vi "Find_calibration_file.vi"(1 "Inst type":T1=enum."Pressure Transducer", 2 "Channel ID":string, 3 "Use Latest Calib":bool, 4 "filename":path) -> (0 "filename out":path)   [LabVIEW 2017]
uses:
  Controls/Inst_type.ctl
  Controls/App_Global.ctl
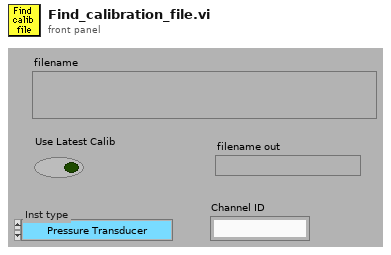
[diagram p1: front panel]
types:
  T1 = typedef "Inst_type.ctl" = enum16{"Propeller anemometer", "Raw voltage", "Pressure Transducer", "Pitot-static tube", "Preston tube", "Hot wire", "Cross wire 1", "Cross wire 2", "Generic Linear", "Generic Polynomial", "Generic BackPoly", "Fast FID", "Thermocouple", "Cold wire", "Pulsed Wire", "LDA Vel", "LDA Tran time", "LDA Arr time", "Microphone"}
  T2 = typedef "App_Global.ctl" = enum16{"Read Global", "Write to Global", "Initialise Array"}
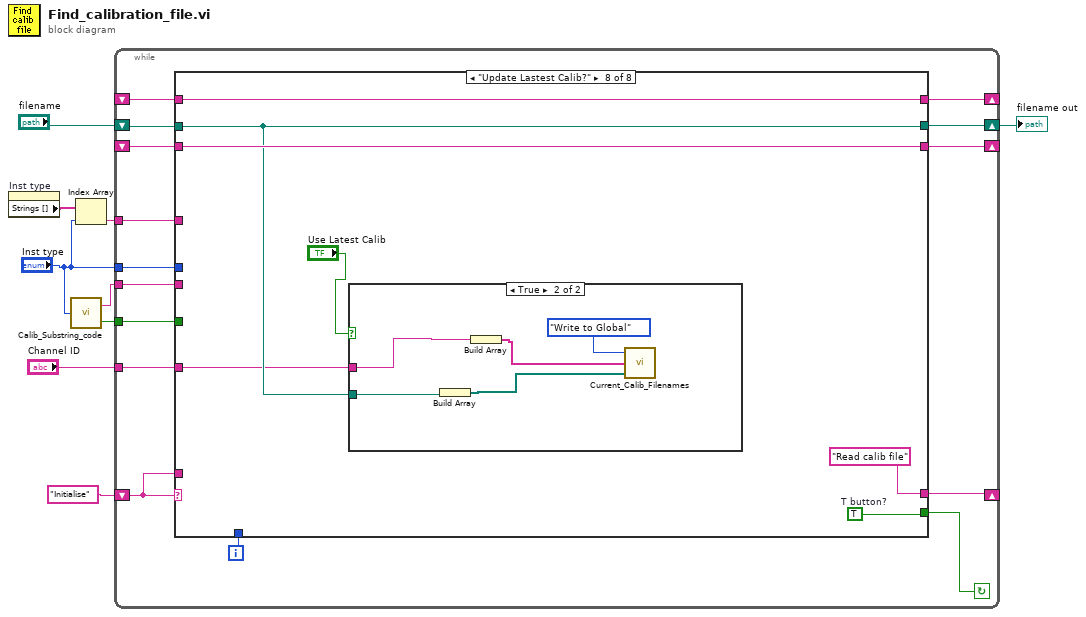
[diagram p0: block diagram]
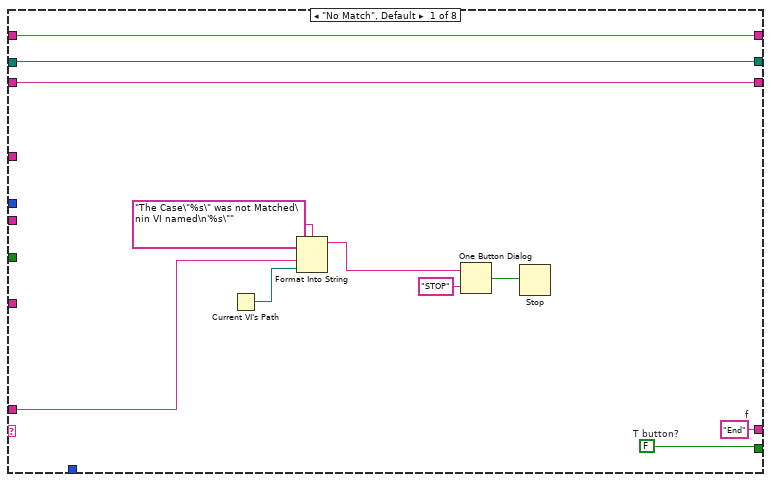
[diagram p2: hidden frame]
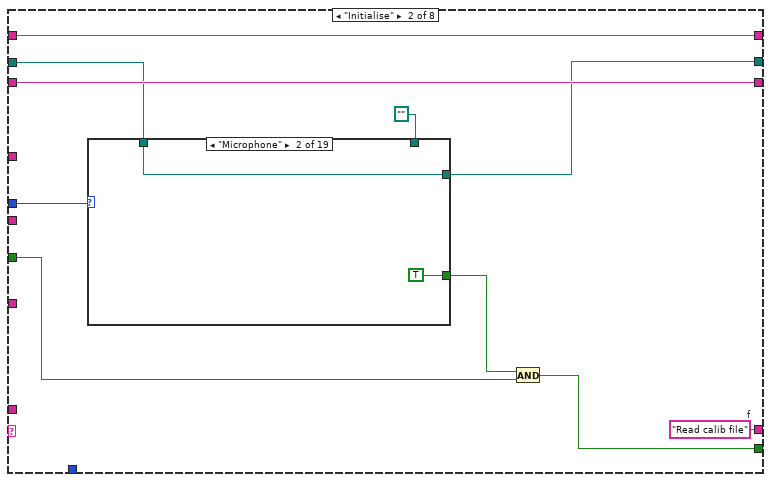
[diagram p3: hidden frame]
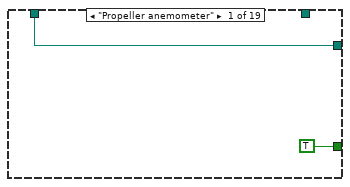
[diagram p4: hidden frame]
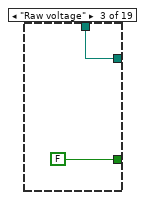
[diagram p5: hidden frame]
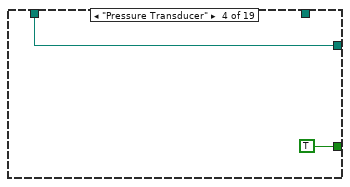
[diagram p6: hidden frame]
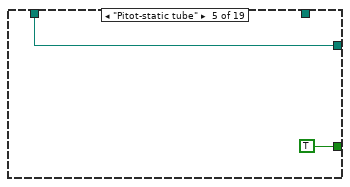
[diagram p7: hidden frame]
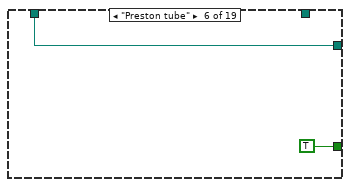
[diagram p8: hidden frame]
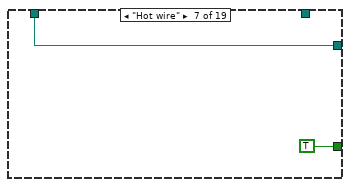
[diagram p9: hidden frame]
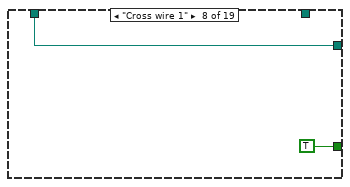
[diagram p10: hidden frame]
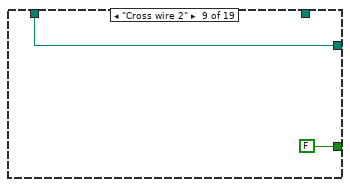
[diagram p11: hidden frame]
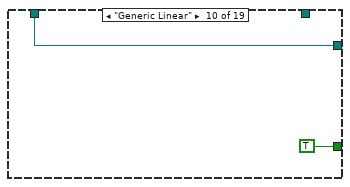
[diagram p12: hidden frame]
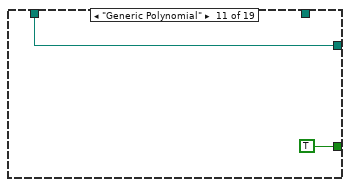
[diagram p13: hidden frame]
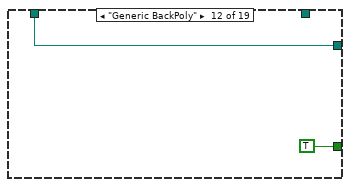
[diagram p14: hidden frame]
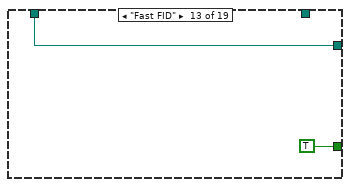
[diagram p15: hidden frame]
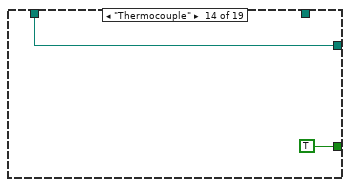
[diagram p16: hidden frame]
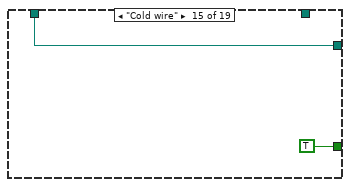
[diagram p17: hidden frame]
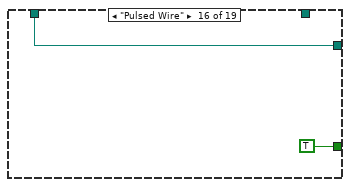
[diagram p18: hidden frame]
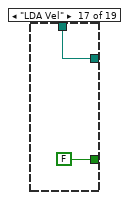
[diagram p19: hidden frame]
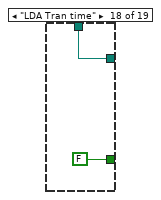
[diagram p20: hidden frame]
diagram:
  n1 = property on="Inst type" class="Enum (strict)"() -> ("Strings []"=w6:string[])  [unwired: 2 in, 2 out]
  n2 = call "Calib_Substring_code.vi"("Inst type"="Inst type") -> ("Substring Type"=w3:string, "Read file"=w2:bool)
  n3 = Index Array(array=w6, index="Inst type") -> (element=w5:string)
  n4 = while {
    shift-left: "filename" -> [w24]
    shift-right: [w23] -> w8
    shift-left: "Initialise" -> [w17]
    shift-right: [w22] -> _
    shift-right: [w19] -> _
    shift-left: _ -> [w18]
    tunnel: "Inst type" -> [w16]
    tunnel: w5 -> [w15]
    shift-right: [w13] -> _
    shift-left: _ -> [w14]
    tunnel: w3 -> [w12]
    tunnel: w2 -> [w11]
    tunnel: "Channel ID" -> [w10]
    i -> [w20]
    stop <- w21 continue-if-true
    n5 = case shown="\"Update Lastest Calib?\"" w17 {
      tunnel: w24 -> [w34 w40 w91 w97 w107 w129 w162 w191]
      tunnel: [w34 w41 w91 w94 w107 w129 w162 w191] -> w23
      tunnel: [w33 w42 w87 "Update Lastest Calib?" w112 w141 "Find a Calibration file" "Read calib file" ("f")] -> w22
      tunnel: [w32 w36 TRUE w103 w115 w142 w177 w189] -> w21
      tunnel: w20 -> [_ _ _ _ _ _ _ _]
      tunnel: [w35 w45 w86 w105 w110 w139 w164 w193] -> w19
      tunnel: w18 -> [w35 w45 _ w105 w110 w139 w164 w193]
      tunnel: w17 -> [w26 _ _ _ _ _ _ _]
      tunnel: w16 -> [_ w43 _ _ _ w140 _ _]
      tunnel: w15 -> [_ _ _ w101 w113 _ _ _]
      tunnel: w14 -> [w25 w44 w84 w102 _ w138 w165 w192]
      tunnel: [w25 w44 w84 w102 w111 w138 w165 w192] -> w13
      tunnel: w12 -> [_ _ _ _ w109 _ _ _]
      tunnel: w11 -> [_ w37 _ _ _ _ _ _]
      tunnel: w10 -> [_ _ _ w99 _ _ _ w188]
      frame "No Match", Default {
        w32 = FALSE  # T button?
        w33 = "End"  # f
        n6 = Current VI's Path() -> (path=w27:path)
        n7 = Format Into String(format string="The Case\"%s\" was not Matched\nin VI named\n'%s\"" ("Format String"), w26, w27) -> (resulting string=w30:string)  [unwired: 2 in, 1 out]
        n8 = One Button Dialog(message=w30, button name ("OK")="STOP") -> (true=w28:bool)
        n9 = Stop(stop? (T)=w28) -> ()
      }
      frame "Initialise" {
        w42 = "Read calib file"  # f
        n10 = case shown="\"Microphone\"" w43 {
          tunnel: [TRUE TRUE FALSE TRUE TRUE TRUE TRUE TRUE FALSE TRUE TRUE TRUE TRUE TRUE TRUE TRUE FALSE FALSE FALSE] -> w38
          tunnel: [w46 w48 w50 w52 w54 w56 w58 w60 w62 w64 w66 w68 w70 w72 w74 w76 w78 w80 w82] -> w41
          tunnel: w40 -> [w46 w48 _ w52 w54 w56 w58 w60 w62 w64 w66 w68 w70 w72 w74 w76 _ _ _]
          tunnel: path "" -> [_ _ w50 _ _ _ _ _ _ _ _ _ _ _ _ _ w78 w80 w82]
          frame "Propeller anemometer" {
          }
          frame "Microphone" {
          }
          frame "Raw voltage" {
          }
          frame "Pressure Transducer" {
          }
          frame "Pitot-static tube" {
          }
          frame "Preston tube" {
          }
          frame "Hot wire" {
          }
          frame "Cross wire 1" {
          }
          frame "Cross wire 2" {
          }
          frame "Generic Linear" {
          }
          frame "Generic Polynomial" {
          }
          frame "Generic BackPoly" {
          }
          frame "Fast FID" {
          }
          frame "Thermocouple" {
          }
          frame "Cold wire" {
          }
          frame "Pulsed Wire" {
          }
          frame "LDA Vel" {
          }
          frame "LDA Tran time" {
          }
          frame "LDA Arr time" {
          }
        }
        n11 = And(x=w38, y=w37) -> (x .and. y?=w36:bool)
      }
      frame "Read calib file" {
        w85 = "Check for calib substring"  # f
        n12 = call "Read_File_Simple.vi"("Filename"=w91) -> ("Error?"=w89:bool, "string"=w86:string)  [unwired: 2 in, 6 out]
        n13 = Select(t="Find a Calibration file", s=w89, f=w85) -> (s? t:f=w87:string)
      }
      frame "Find a Calibration file" {
        n14 = Format Into String(format string=" calibration file for channel %s not found.  Please search for it.", initial string=w101, w99) -> (resulting string=w93:string)  [unwired: 1 in, 1 out]
        n15 = call "Current_Filepath.vi"("Short_Name"="Cal" ("Data Type"), "Filename in"=w97, "Data Type"="Calibrations") -> ("Directory"=w96:path)  [unwired: 1 in, 1 out]
        n16 = call "File Dialog"("start path"=w96, "prompt"=w93) -> ("selected path"=w94:path, "cancelled"=w95:bool)  [unwired: 10 in, 2 out]
        n17 = Not(x=w95) -> (.not. x?=w103:bool)
      }
      frame "Check for calib substring" {
        w117 = FALSE  # Show Dialog?
        n18 = Concatenate Strings(w109, "calib label") -> (w114:string)
        n19 = Format Into String(format string="Calibration File   %s", w107) -> (resulting string=w106:string)  [unwired: 2 in, 1 out]
        n20 = call "Get_string_subset.vi"("String Name"=w106, "Show Dialog?"=w117, "String to split"=w110, "File Label"=w114) -> ("Status"=w116:enum16{"Char in string", "Char not in string"}, "Output string"=w111:string)
        n21 = case shown="\"Char in string\"" w116 {
          tunnel: [TRUE w126] -> w115
          tunnel: w107 -> [_ w122]
          tunnel: w113 -> [_ w125]
          tunnel: ["Was there sufficient calibration points?" "Find a Calibration file"] -> w112
          frame "Char in string" {
          }
          frame "Char not in string" {
            w123 = "The calibration file\n\"%s\"\nis not the appropriate file for a %s"  # format string
            w127 = "Find another file"  # T button name ("OK")
            n22 = Strip Path(path=w122) -> (name=w121:string)  [unwired: 1 out]
            n23 = Format Into String(format string=w123, w121, w125) -> (resulting string=w128:string)  [unwired: 2 in, 1 out]
            n24 = Two Button Dialog(message=w128, 2:w127) -> (T button?=w126:bool)  [unwired: 1 out]
          }
        }
      }
      frame "Was there sufficient calibration points?" {
        n25 = Format Into String(format string="Calibration File   %s", w129) -> (resulting string=w130:string)  [unwired: 2 in, 1 out]
        n26 = call "2D_array_from_string.vi"("String Name"=w130, "Input string"=w138, "Array title"="Calib points label") -> ("2D data array"=w137:dbl[][])  [unwired: 1 in]
        n27 = for {
          tunnel: w137 -> [w148] mode=indexing
          tunnel: [w144] -> w133 mode=indexing
          n28 = Index Array(array=w148, index=5) -> (element=w146:dbl)
          n29 = Not A Number/Path/Refnum?(number/path/refnum=w146) -> (NaN/Path/Refnum?=w145:bool)
          n30 = Not(x=w145) -> (.not. x?=w144:bool)
        }
        n31 = Boolean To (0,1)(Boolean=w133) -> (0, 1=w136:i16[])
        n32 = Add Array Elements(numeric array=w136) -> (sum=w134:i16)
        n33 = Greater?(x=w134, y=i16 1) -> (0:w132:bool)
        n34 = case shown="True" w132 {
          tunnel: [w153 w157] -> w142
          tunnel: w129 -> [w150 _]
          tunnel: ["Find a Calibration file" "Are XW psi 1 and 2 valid"] -> w141
          tunnel: w140 -> [_ w158]
          frame False {
            w151 = "The calibration file\n\"%s\"\nhas less than two calibration points."  # format string
            w154 = "Find another file"  # T button name ("OK")
            n35 = Strip Path(path=w150) -> (name=w149:string)  [unwired: 1 out]
            n36 = Format Into String(format string=w151, w149) -> (resulting string=w155:string)  [unwired: 2 in, 1 out]
            n37 = Two Button Dialog(message=w155, 2:w154) -> (T button?=w153:bool)  [unwired: 1 out]
          }
          frame True {
            n38 = case shown="\"Propeller anemometer\", Default" w158 {
              tunnel: [FALSE TRUE] -> w157
              frame "Propeller anemometer", Default {
              }
              frame "Cross wire 1" {
              }
            }
          }
        }
      }
      frame "Are XW psi 1 and 2 valid" {
        w170 = FALSE  # Show Dialog?
        n39 = Build Array("C0", "C1", "C2") -> (w172:string[])
        n40 = Format Into String(format string="Calibration File   %s", w162) -> (resulting string=w161:string)  [unwired: 2 in, 1 out]
        n41 = call "Get_string_subset.vi"("String Name"=w161, "Show Dialog?"=w170, "String to split"=w164, "File Label"="Auxiliary constants") -> ("Output string"=w171:string)  [unwired: 1 out]
        n42 = for {
          tunnel: w172 -> [w180] mode=indexing
          tunnel: [w179] -> w169 mode=indexing
          tunnel: w171 -> [w178]
          n43 = call "Get_value_from_string.vi"("Input string"=w178, "Variable name"=w180) -> ("Value"=w179:dbl)  [unwired: 1 in, 1 out]
        }
        n44 = Not A Number/Path/Refnum?(number/path/refnum=w169) -> (NaN/Path/Refnum?=w168:bool[])
        n45 = Or Array Elements(Boolean array=w168) -> (logical OR=w167:bool)
        n46 = case shown="False" w167 {
          tunnel: [FALSE w185] -> w177
          tunnel: w162 -> [_ w183]
          frame False {
          }
          frame True {
            n47 = Strip Path(path=w183) -> (name=w182:string)  [unwired: 1 out]
            n48 = Format Into String(format string="The XW calibration file\n\"%s\"\ndoes not have valid angle calibration coefficients.", w182) -> (resulting string=w187:string)  [unwired: 2 in, 1 out]
            n49 = Two Button Dialog(message=w187, 2:"Find another file" ("T button name (\"OK\")")) -> (T button?=w185:bool)  [unwired: 1 out]
          }
        }
      }
      frame "Update Lastest Calib?" {
        w189 = TRUE  # T button?
        n50 = case shown="True" "Use Latest Calib" {
          tunnel: w191 -> [_ w198]
          tunnel: w188 -> [_ w195]
          frame False {
          }
          frame True {
            n51 = Build Array(w198) -> (w196:path[])
            n52 = Build Array(w195) -> (w197:string[])
            n53 = call "Current_Calib_Filenames.vi"("Calib Filename"=w196, "Channel ID input"=w197, "Mode"=App_Global."Write to Global") -> ()  [unwired: 3 out]
          }
        }
      }
    }
  }
  "filename out" <- w8
